vi "e.gate HighSpeedPort Online Communication.vi"(5 "ReadCount":i32, 6 "ValueArray":dbl[](array[numeric]), 7 "ReadIndex":i32, 8 "error in (no error)":errorcluster, 9 "WriteCount":i32, 10 "WriteIndex":i32, 11 "e.gate Configuration In":T1) -> (0 "error out":errorcluster, 2 "Value":dbl[](array[numeric]), 3 "e.gate Configuration Out":T1)   [LabVIEW 2016]
doc: "<B>AMC - Analytik & Messtechnik GmbH Chemnitz</B>\n\nLabVIEW Drivers for e.gate / e.pac series from Gantner Instruments\n\nThis VI reads a value specified by <B>Channel</B> from a device specified by <B>connection ID In</B>."
uses:
  e.gate Configuration.ctl
  e.gate Channel Data.ctl
  e.gate Data Type.ctl
  e.gate Protocol Type.ctl
  e.gate Module  Data.ctl
  e.gateHSP_DLLhandle.ctl
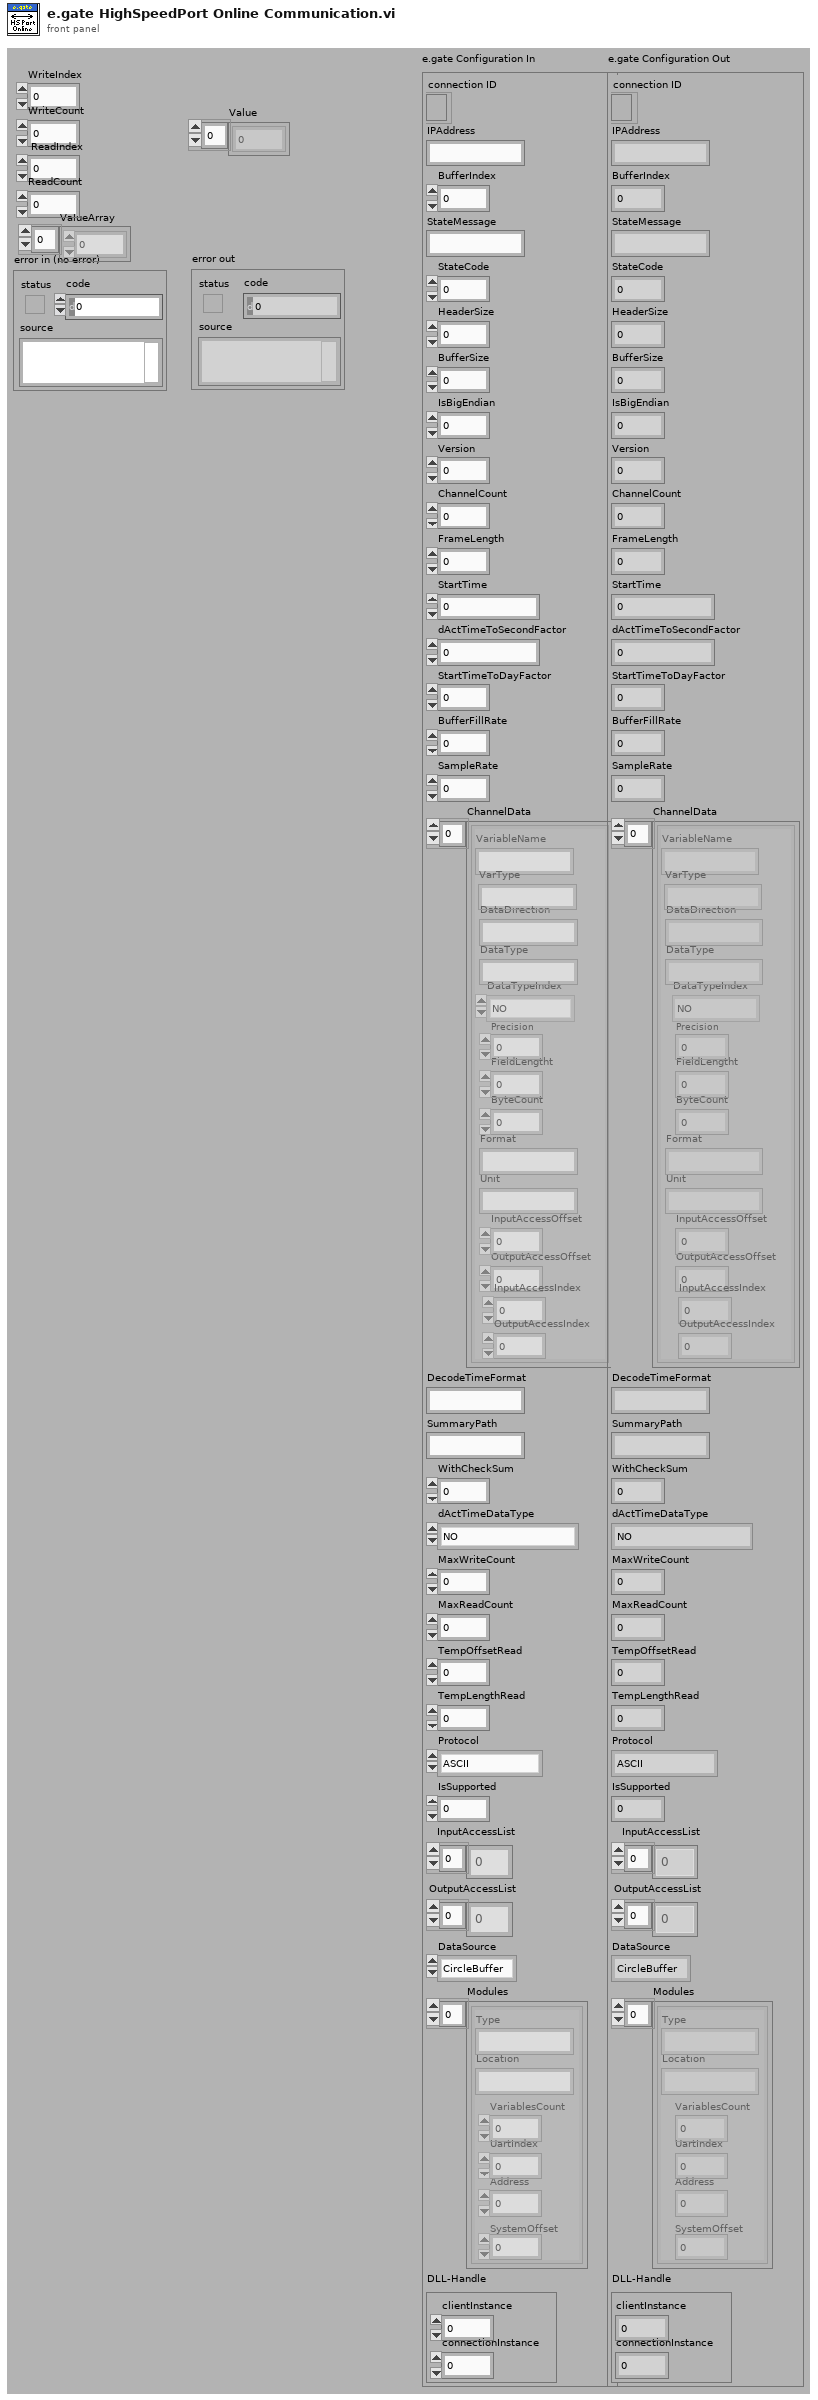
[diagram p1: front panel]
types:
  T1 = typedef "e.gate Configuration.ctl" = cluster{"connection ID":refnum<k5>, "IPAddress":string, "BufferIndex":i32, "StateMessage":string, "StateCode":i8, "HeaderSize":i32, "BufferSize":i32, "IsBigEndian":i32, "Version":i32, "ChannelCount":i32, "FrameLength":i32, "StartTime":dbl, "dActTimeToSecondFactor":dbl, "StartTimeToDayFactor":dbl, "BufferFillRate":dbl, "SampleRate":dbl, "ChannelData":T2[], "DecodeTimeFormat":string, "SummaryPath":string, "WithCheckSum":i32, "dActTimeDataType":T3, "MaxWriteCount":i32, "MaxReadCount":i32, "TempOffsetRead":i32, "TempLengthRead":i32, "Protocol":T4, "IsSupported":i32, "InputAccessList":i32[], "OutputAccessList":i32[], "DataSource":enum16{"CircleBuffer", "test.con Logger", "test.con Archive"}, "Modules":T5[], "DLL-Handle":T6}
  T2 = typedef "e.gate Channel Data.ctl" = cluster{"VariableName":string, "DataDirection":string, "DataType":string, "DataTypeIndex":T3, "Precision":i16, "FieldLengtht":i16, "ByteCount":i32, "Format":string, "Unit":string, "InputAccessOffset":i32, "OutputAccessOffset":i16, "InputAccessIndex":i16, "OutputAccessIndex":i16, "VarType":string}
  T3 = typedef "e.gate Data Type.ctl" = enum16{"NO", "BOOL", "SINT8", "USINT8", "SINT16", "USINT16", "SINT32", "USINT32", "FLOAT", "SET8", "SET16", "SET32", "DOUBLE", "SINT64", "USINT64", "SET64"}
  T4 = typedef "e.gate Protocol Type.ctl" = enum16{"ASCII", "HighspeedPort Online", "HighspeedPort Buffer", "eGateHighspeedPortDLL "}
  T5 = typedef "e.gate Module  Data.ctl" = cluster{"Type":string, "Location":string, "VariablesCount":i16, "UartIndex":i16, "Address":i16, "SystemOffset":i16}
  T6 = typedef "e.gateHSP_DLLhandle.ctl" = cluster{"clientInstance":i32, "connectionInstance":i32}
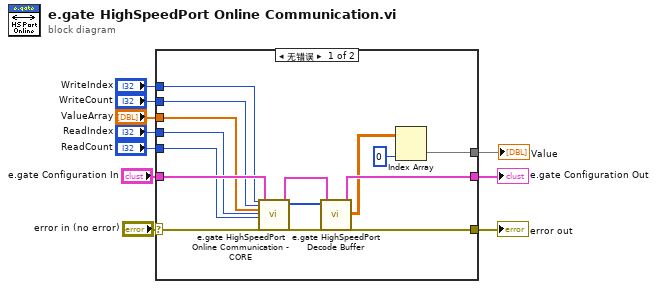
[diagram p0: block diagram]
diagram:
  n1 = case shown="无错误" "error in (no error)" {
    selector: "error in (no error)" -> [w24 w27]
    tunnel: "e.gate Configuration In" -> [w25 w26]
    tunnel: [w21 w26] -> w8
    tunnel: [w20 w27] -> w7
    tunnel: [w17 _] -> w6
    tunnel: "WriteIndex" -> [w16 _]
    tunnel: "WriteCount" -> [w15 _]
    tunnel: "ValueArray" -> [w14 _]
    tunnel: "ReadIndex" -> [w13 _]
    tunnel: "ReadCount" -> [w12 _]
    frame No Error {
      n2 = call "e.gate HighSpeedPort Online Communication - CORE.vi"("WriteIndex"=w16, "WriteCount"=w15, "ValueArray"=w14, "ReadIndex"=w13, "ReadCount"=w12, "error in (no error)"=w24, "Configuration in"=w25) -> ("Configuration out"=w22:T1, "data array (binary)"=w19:u8[], "error out"=w23:errorcluster)  [unwired: 18 out]
      n3 = call "e.gate HighSpeedPort Decode Buffer.vi"("Data in (binary)"=w19, "error in"=w23, "Configuration  in"=w22) -> ("Configuration out"=w21:T1, "data array (double)"=w18:dbl[][], "error out"=w20:errorcluster)  [unwired: 1 in, 21 out]
      n4 = Index Array(array=w18, index (col)=0 ("index (row)")) -> (element=w17:dbl[])  [unwired: 1 in]
    }
    frame Error {
    }
  }
  "error out" <- w7
  "e.gate Configuration Out" <- w8
  "Value" <- w6
